vi "Connect_LTA-HS.vi"(8 "error in (no error)":errorcluster, 11 "VISA resource name":refnum<visa-resource-name>) -> (0 "error out (duplicate)":errorcluster, 3 "Device Connection Cluster":T1)   [LabVIEW 2013]
panel:
  out "Interface Information:Interface Number":u16
  out "General Settings:Resource Name":string
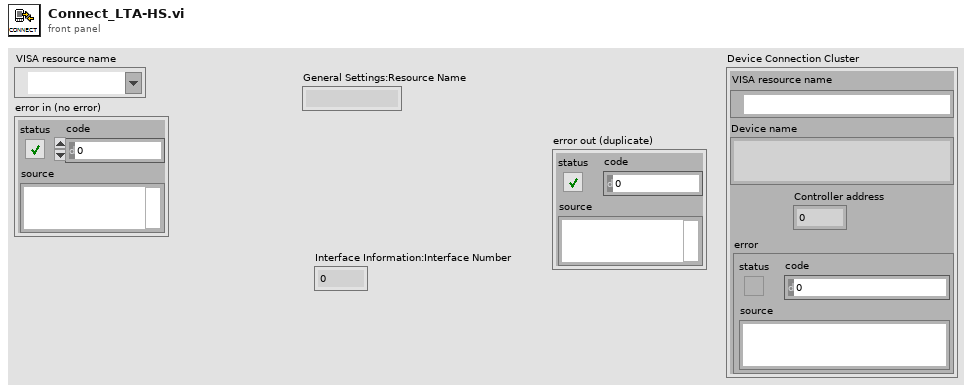
[diagram p1: front panel]
types:
  T1 = cluster{"VISA resource name":refnum<visa-resource-name>, "Device name":string, "Controller address":i32, "error":errorcluster}
  T2 = cluster{"input XON/XOFF":bool, "input HW Handshake":bool, "input alt HW HShk":bool, "output XON/XOFF":bool, "output HW Handshake":bool, "output alt HW HShk":bool, "XOFF byte ":u8, "XON byte":u8, "parity error byte":u16}
  T3 = cluster{"VISA resource name":refnum<visa-resource-name>, string, i32, "error out":errorcluster}
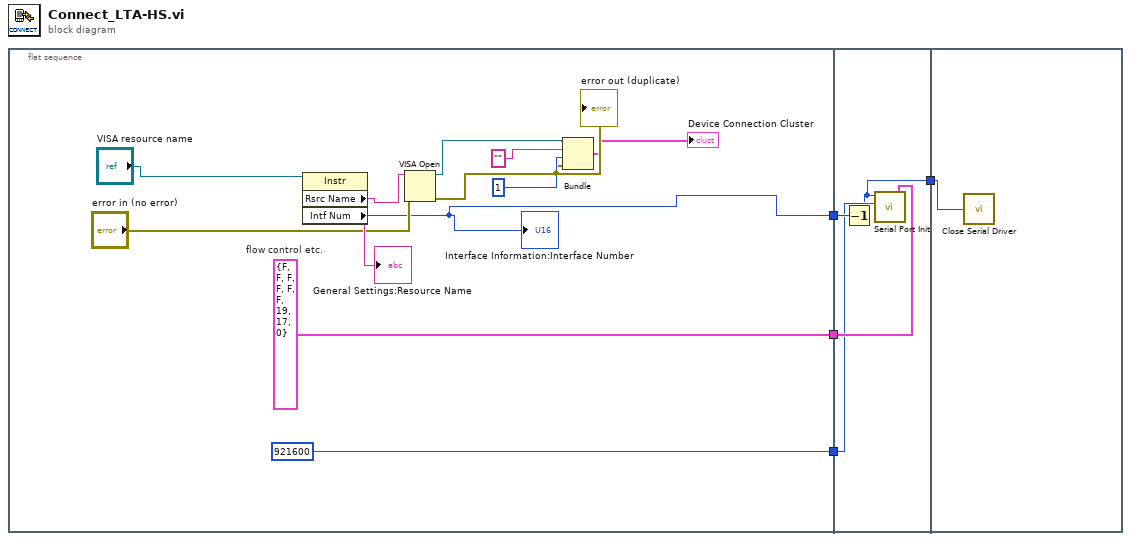
[diagram p0: block diagram]
diagram:
  n1 = flat-sequence {
    tunnel: [w7] -> w4
    tunnel: [w6] -> w3
    tunnel: [u32 921600 ("baud rate")] -> w2
    tunnel: w4 -> [w19]
    tunnel: w3 -> [w18]
    tunnel: w2 -> [w17]
    tunnel: [w16] -> w1
    tunnel: w1 -> [w20]
    frame #0 {
      w6 = T2 {"input XON/XOFF"=FALSE, "input HW Handshake"=FALSE, "input alt HW HShk"=FALSE, "output XON/XOFF"=FALSE, "output HW Handshake"=FALSE, "output alt HW HShk"=FALSE, "XOFF byte "=19, "XON byte"=17, "parity error byte"=0}  # flow control etc.
      n2 = property class="Instr"(reference="VISA resource name") -> ("Rsrc Name"=w14:string, "Intf Num"=w7:u16)  [unwired: 1 in, 2 out]
      "General Settings:Resource Name" <- w14
      "Interface Information:Interface Number" <- w7
      n3 = VISA Open(error in (no error)="error in (no error)", VISA resource name=w14) -> (VISA resource name=w13:refnum<visa-resource-name>, error out=w10:errorcluster)  [unwired: 3 in]
      "error out (duplicate)" <- w10
      n4 = Bundle("VISA resource name"=w13, "", 1, "error out"=w10) -> (→"Device Connection Cluster":T3)  [unwired: 1 in]
    }
    frame #1 {
      n5 = Decrement(x=w19) -> (x-1=w16:u16)
      n6 = call <vilib>:"Serial Port Init.vi"("flow control etc."=w18, "baud rate"=w17, "port number"=w16) -> ()  [unwired: 4 in, 1 out]
    }
    frame #2 {
      n7 = call <vilib>:"Close Serial Driver.vi"("port number"=w20) -> ()  [unwired: 1 out]
    }
  }
